vi "Value by Index.vi"(8 "error in (no error)":errorcluster, 10 "Index":i32, 11 "Group in":refnum<class "Group.lvclass">) -> (0 "error out":errorcluster, 1 "Timestamp":dbl, 2 "Scaled":dbl, 3 "Group out":refnum<class "Group.lvclass">, 4 "Raw":dbl)   [LabVIEW 2020, in "Vecto.lvlib" / "Group.lvclass"]
uses:
  Group.lvclass
  Group.lvclass/Group.ctl
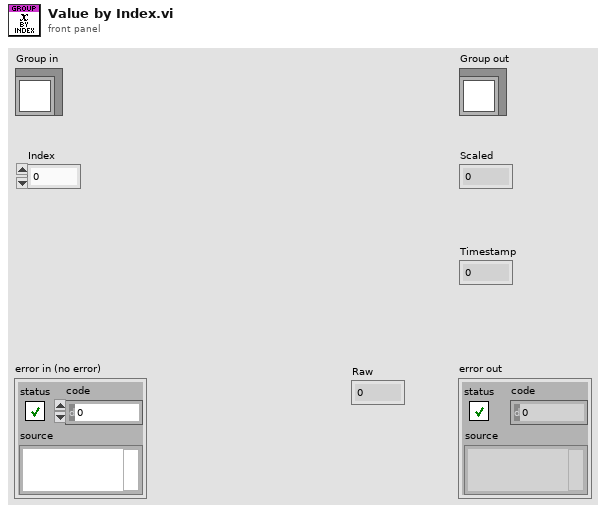
[diagram p1: front panel]
types:
  T1 = typedef "Vecto.lvlib/Group.lvclass/Ref.ctl" = cluster{"Channel Index Map":map{string, i32}, "Channel Info":T2[], "Scaled":dbl[], "Timestamp":dbl[], "Raw":dbl[]}
  T2 = typedef "Vecto.lvlib/Channel Info.ctl" = cluster{"Name":string, "Group":string, "Owning Node":u32, "Owning Task":u32, "Resource":string}
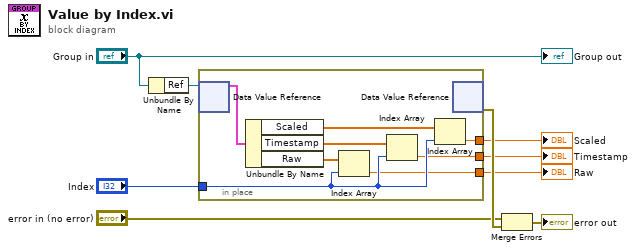
[diagram p0: block diagram]
diagram:
  n1 = Unbundle By Name("Group in") -> ("Ref"=w7:refnum<data-value>)
  n2 = in-place {
    in-place-border: "Index" -> [w13]
    in-place-border: [w12] -> w2
    in-place-border: [w11] -> w3
    in-place-border: [w10] -> w4
    n3 = in-place-dvr #1(w7) -> (w17:T1)  [unwired: 1 out]
    n4 = Unbundle By Name(w17) -> ("Scaled"=w14:dbl[], "Timestamp"=w15:dbl[], "Raw"=w16:dbl[])
    n5 = Index Array(array=w16, index=w13) -> (element=w12:dbl)
    n6 = Index Array(array=w15, index=w13) -> (element=w11:dbl)
    n7 = Index Array(array=w14, index=w13) -> (element=w10:dbl)
    n8 = in-place-dvr #1() -> (w9:errorcluster)  [unwired: 1 in, 1 out]
  }
  "Scaled" <- w4
  "Timestamp" <- w3
  "Raw" <- w2
  n9 = Merge Errors("error in (no error)", w9) -> (→"error out":errorcluster)
  "Group out" <- "Group in"
